vi "IsCallerHasAccess.vi"(8 "error in (no error)":errorcluster, 11 "Topas":refnum<k24>) -> (0 "error out":errorcluster, 2 "GetCallerHasAccess":bool, 3 "Topas out":refnum<k24>)   [LabVIEW 2017]
uses:
  D:/upwork/Laser Measurement Tool/Topas4PublicAPI/NET_SDK/Topas4Lib.dll
  Topas4PublicAPI/NET_SDK/Topas4Lib.dll
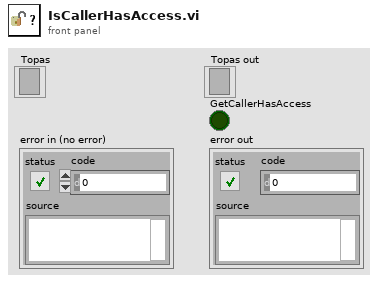
[diagram p1: front panel]
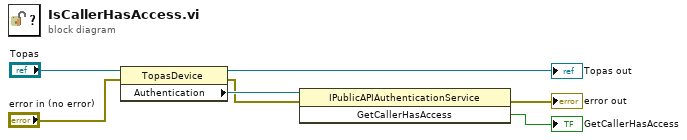
[diagram p0: block diagram]
diagram:
  n1 = property class="TopasDevice"(reference="Topas", error in="error in (no error)") -> (reference out=→"Topas out":refnum<k24>, error out=w4:errorcluster, "Authentication"=w5:refnum<k24>)
  n2 = invoke class="IPublicAPIAuthenticationService" method="GetCallerHasAccess"(reference=w5, error in=w4) -> (error out=→"error out":errorcluster, "GetCallerHasAccess"=→"GetCallerHasAccess":bool)  [unwired: 1 in, 1 out]
